vi "Clear Index.vi"(8 "error in (no error)":errorcluster) -> (0 "error out":errorcluster)   [LabVIEW 2020, in "Test Finder.lvclass"]
uses:
  Test Finder.lvclass
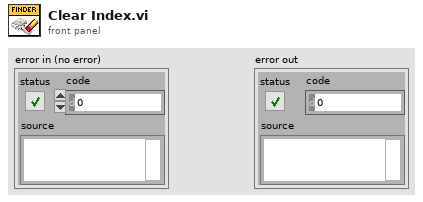
[diagram p1: front panel]
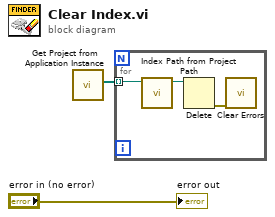
[diagram p0: block diagram]
diagram:
  n1 = call "Get Project from Application Instance.vi"() -> ("Open Projects"=w1:path[])  [unwired: 10 in, 1 out]
  n2 = for {
    tunnel: w1 -> [w3] mode=indexing
    n3 = call "Index Path from Project Path.vi"("Project Path"=w3) -> ("appended path"=w5:path)  [unwired: 10 in]
    n4 = Delete(path (use dialog)=w5) -> (error out=w4:errorcluster)  [unwired: 4 in, 2 out]
    n5 = call <vilib>:"Clear Errors.vi"("error in (no error)"=w4) -> ()  [unwired: 5 in, 2 out]
  }
  "error out" <- "error in (no error)"
